vi "Betonauswahl.vi"(8 "error in (no error)":errorcluster) -> (0 "error out":errorcluster)   [LabVIEW 2023]
doc: "Dieses VI ließt das config file für die betonsorten und errechnet den preis pro menge \nerstellt: Stojanovic Sara\nDatum: 12.11.2025"
uses:
  CONTROLS/Betonauswahl.ctl
  <vilib>/Utility/miscctls.llb/LVRectTypeDef.ctl
panel:
  out "Preis":dbl
  in  "Betonauswahl":T1
  in  "Menge (in m3)":dbl
  in  "Reserve Schalter 3":bool
  in  "Reserve Schalter 2":bool
  in  "Reserve Schalter":bool
  in  "Daten speichern":bool
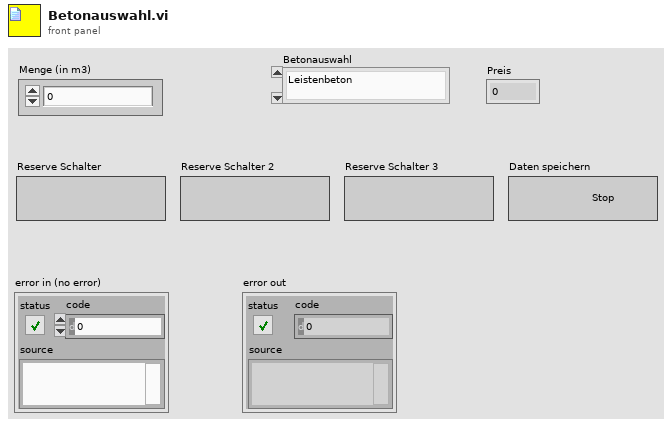
[diagram p1: front panel]
types:
  T1 = typedef "Betonauswahl.ctl" = enum16{"Leistenbeton", "Erdfeuchterbeton", "Beton", "Erdfeuchter starker Beton", "Starker Beton"}
  T2 = typedef "LVRectTypeDef.ctl" = cluster{"Left":i16, "Top":i16, "Right":i16, "Bottom":i16}
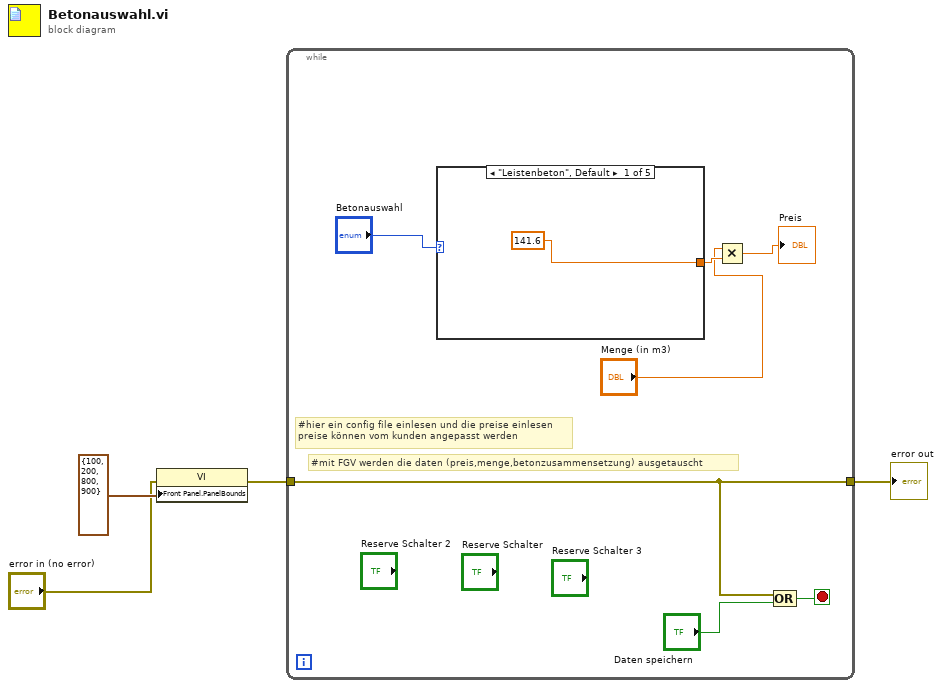
[diagram p0: block diagram]
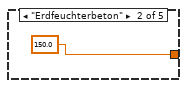
[diagram p2: hidden frame]
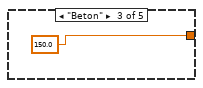
[diagram p3: hidden frame]
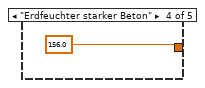
[diagram p4: hidden frame]
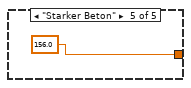
[diagram p5: hidden frame]
diagram:
  n1 = property class="VI"(error in="error in (no error)", "Front Panel.PanelBounds"=T2 {"Left"=100, "Top"=200, "Right"=800, "Bottom"=900} ("Front Panel Window:Panel Bounds")) -> (error out=w1:errorcluster)  [unwired: 1 in, 1 out]
  n2 = while {
    tunnel: [w10] -> w4
    tunnel: w1 -> [w10]
    stop <- w9 stop-if-true
    # "#mit FGV werden die daten (preis,menge,betonzusammensetzung) ausgetauscht"
    # "#hier ein config file einlesen und die preise einlesen\npreise können vom kunden angepasst werden"
    n3 = case shown="\"Leistenbeton\", Default" "Betonauswahl" {
      tunnel: [141.6 150.0 150.0 156.0 156.0] -> w7
      frame "Leistenbeton", Default {
      }
      frame "Erdfeuchterbeton" {
      }
      frame "Beton" {
      }
      frame "Erdfeuchter starker Beton" {
      }
      frame "Starker Beton" {
      }
    }
    n4 = Multiply(x="Menge (in m3)", y=w7) -> (x*y=→"Preis":dbl)
    n5 = Compound Arithmetic op=OR(w10, "Daten speichern") -> (w9:bool)
  }
  "error out" <- w4
